vi "ddsTimeArrayConvert.vi"(7 "Pre 3.0 AOM driver version?":bool, 10 "Register":dbl=10.0 min=0.0 max=15.0 step=1.0 format="%#.1f", 11 "Time Array (ms)":dbl[](array[numeric])=[0.0] min=0.0 max=42000.0 step=1e-05 format="%.5f") -> (3 "Characters for FPGA":string="L:00000000\r\n")   [LabVIEW 2013, in "DDS9954_v2013.lvlib"]
uses:
  DDS9954_v2013.lvlib
  dataToAscii_32bit.vi
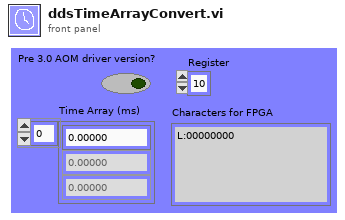
[diagram p1: front panel]
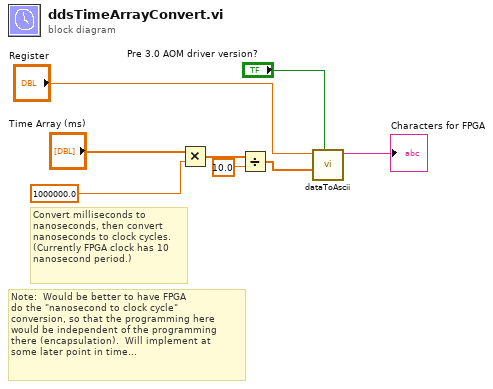
[diagram p0: block diagram]
diagram:
  # "Note:  Would be better to have FPGA\ndo the \"nanosecond to clock cycle\" \nconversion, so that the programming here\nwould be independent of the programming \nthere (encapsulation).  Will implement at \nsome later point in time..."
  # "Convert milliseconds to\nnanoseconds, then convert\nnanoseconds to clock cycles.\n(Currently FPGA clock has 10\nnanosecond period.)"
  n1 = Multiply(x="Time Array (ms)", y=1000000.0) -> (x*y=w6:dbl[])
  n2 = Divide(x=w6, y=10.0) -> (x/y=w2:dbl[])
  n3 = call-poly "dataToAscii.vi"("Pre 3.0 AOM driver version?"="Pre 3.0 AOM driver version?", "Input Data"=w2, "Register"="Register") -> ("Characters to FPGA"=→"Characters for FPGA":string)  [unwired: 8 in]
